vi "Initialise.vi"(8 "error in (no error)":errorcluster, 11 "TDMS Sink in":refnum<class "TDMS Sink.lvclass">) -> (0 "error out":errorcluster, 3 "TDMS Sink out":refnum<class "TDMS Sink.lvclass">)   [LabVIEW 2020, in "LV Log.lvlib" / "TDMS Sink.lvclass"]
uses:
  TDMS Sink.lvclass
  TDMS Sink.lvclass/TDMS Sink.ctl
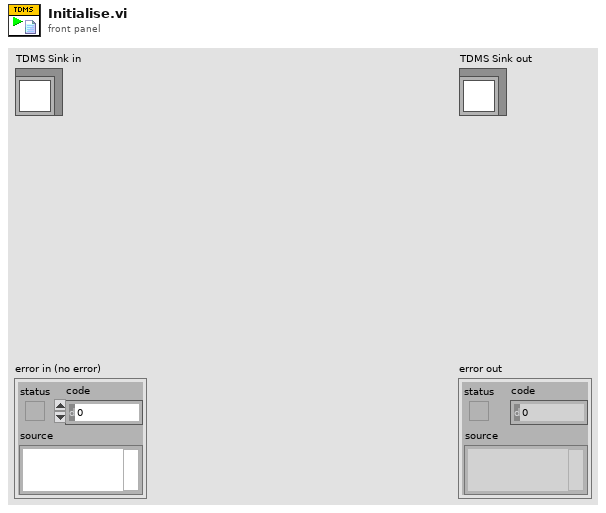
[diagram p1: front panel]
types:
  T1 = enum16{"open", "open or create", "create or replace", "create", "open (read-only)"}
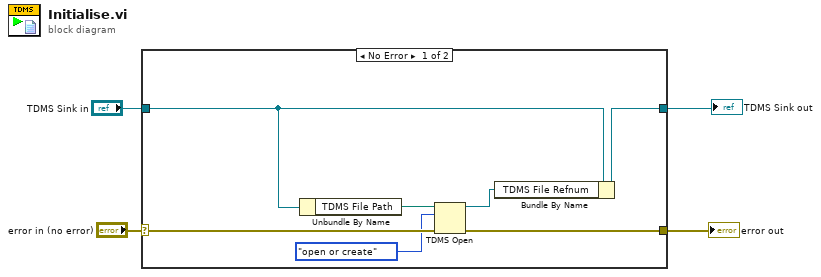
[diagram p0: block diagram]
diagram:
  n1 = case shown="No Error" "error in (no error)" {
    selector: "error in (no error)" -> [w10 w13]
    tunnel: [w9 w13] -> w1
    tunnel: [w11 w12] -> w3
    tunnel: "TDMS Sink in" -> [w6 w12]
    frame No Error {
      n2 = Unbundle By Name(w6) -> ("TDMS File Path"=w5:path)
      n3 = TDMS Open(8:w10, 10:T1."open or create" ("operation (0:open)"), 11:w5) -> (0:w9:errorcluster, 3:w7:refnum<k34>)  [unwired: 4 in]
      n4 = Bundle By Name(cluster=w6, "TDMS File Refnum"=w7) -> (w11:refnum<class "TDMS Sink.lvclass">)
    }
    frame Error {
    }
  }
  "error out" <- w1
  "TDMS Sink out" <- w3
